vi "Kill Symbol Map Daemon.vi"(8 "error in (no error)":errorcluster, 11 "TwinCAT ADS in":refnum<class "TwinCAT ADS.lvclass">) -> (0 "error out":errorcluster, 3 "TwinCAT ADS out":refnum<class "TwinCAT ADS.lvclass">)   [LabVIEW 2018, in "TwinCAT ADS.lvclass"]
uses:
  TwinCAT ADS.lvclass
  TwinCAT ADS.lvclass/TwinCAT ADS.ctl
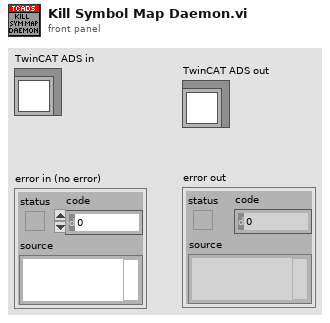
[diagram p1: front panel]
types:
  T1 = typedef "TwinCAT ADS.lvclass/Daemon Message.ctl" = cluster{"Symbol Name":string, "Occurrence":refnum<k4>}
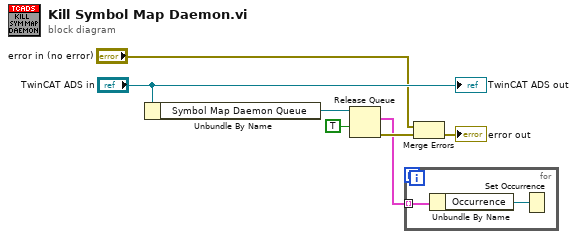
[diagram p0: block diagram]
diagram:
  n1 = Unbundle By Name("TwinCAT ADS in") -> ("Symbol Map Daemon Queue"=w3:refnum<queue>)
  n2 = Release Queue(queue=w3, force destroy? (F)=TRUE) -> (remaining elements=w1:T1[], error out=w6:errorcluster)  [unwired: 1 in, 1 out]
  n3 = for {
    tunnel: w1 -> [w9] mode=indexing
    n4 = Unbundle By Name(w9) -> ("Occurrence"=w8:refnum<k4>)
    n5 = Set Occurrence(w8) -> ()
  }
  n6 = Merge Errors("error in (no error)", w6) -> (→"error out":errorcluster)
  "TwinCAT ADS out" <- "TwinCAT ADS in"
